vi "JAS-Color Sensor V3 Match Color.vi"(11 "Measured Color":cluster{"R":dbl, "G":dbl, "B":dbl}) -> (1 "Confidence":dbl, 2 "Matched Color":cluster{"R":dbl, "G":dbl, "B":dbl}, 3 "Matched Color Name":string)   [LabVIEW 2019]
uses:
  JAS-ColorMatch-FGV-Cmd.ctl
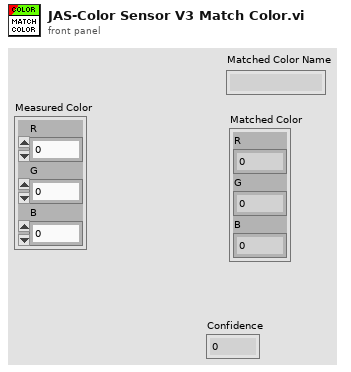
[diagram p1: front panel]
types:
  T1 = typedef "JAS-ColorMatch-FGV-Cmd.ctl" = enum16{"AddNew", "Update", "Read"}
  T2 = typedef "Color Sensor V3 Color Match.ctl" = cluster{"Name":string, "Normalized Color":cluster{"R":dbl, "G":dbl, "B":dbl}}
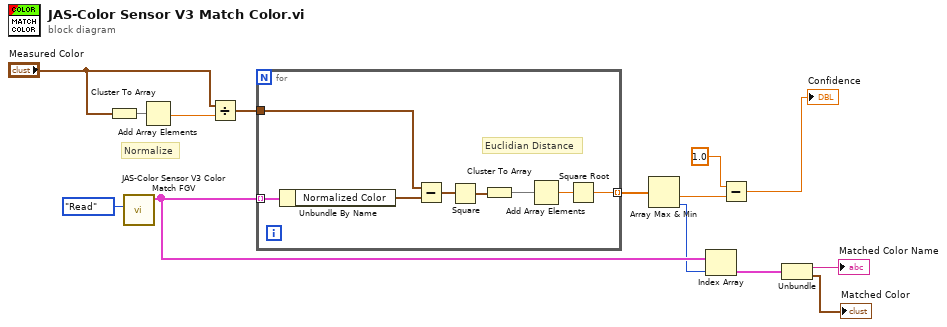
[diagram p0: block diagram]
diagram:
  # "Normalize"
  n1 = Cluster To Array(cluster="Measured Color") -> (array=w5:dbl[])
  n2 = call "JAS-Color Sensor V3 Color Match FGV.vi"("ColorMatchFGV-Cmd"=JAS-ColorMatch-FGV-Cmd."Read") -> ("All Match Colors"=w10:T2[])  [unwired: 9 in, 1 out]
  n3 = Add Array Elements(numeric array=w5) -> (sum=w4:dbl)
  n4 = Divide(x="Measured Color", y=w4) -> (x/y=w2:cluster{"R":dbl, "G":dbl, "B":dbl})
  n5 = for {
    tunnel: w10 -> [w22] mode=indexing
    tunnel: w2 -> [w21]
    tunnel: [w15] -> w14 mode=indexing
    # "Euclidian Distance"
    n6 = Unbundle By Name(w22) -> ("Normalized Color"=w20:cluster{"R":dbl, "G":dbl, "B":dbl})
    n7 = Subtract(x=w21, y=w20) -> (x-y=w19:cluster{"R":dbl, "G":dbl, "B":dbl})
    n8 = Square(x=w19) -> (x^2=w18:cluster{"R":dbl, "G":dbl, "B":dbl})
    n9 = Cluster To Array(cluster=w18) -> (array=w17:dbl[])
    n10 = Add Array Elements(numeric array=w17) -> (sum=w16:dbl)
    n11 = Square Root(x=w16) -> (sqrt(x)=w15:dbl)
  }
  n12 = Array Max & Min(array=w14) -> (min value=w13:dbl, min index (indices)=w9:i32)  [unwired: 2 out]
  n13 = Index Array(array=w10, index=w9) -> (element=w8:T2)
  n14 = Subtract(x=1.0 ("max value"), y=w13) -> (x-y=→"Confidence":dbl)
  n15 = Unbundle(w8) -> ("Name"=→"Matched Color Name":string, "Normalized Color"=→"Matched Color":cluster{"R":dbl, "G":dbl, "B":dbl})
